vi "calculate_parameters.vi"(10 "Experimental Variables":T2={"Pixel Size before binning (µm)"=14.2, "Imaging Wavelength (m)"=4.61e-07, "Isotope"=84, "1P1 Linewidth (MHz)"=32.0, "Imaging Detuning (MHz)"=0.0, "Software Bin Size"=1, "Exp. Trigger ON time (ms)"=0.0, "Path to spinapi.dll"=path "C:/SpinCore/SpinAPI/lib32/spinapi.dll", "PB clock_freq (MHz)"=100.0} {"Software Bin Size" items=["1"=1, "2"=2, "3"=3, "4"=4, "5"=5, "6"=6, "7"=7, "8"=8]; "Isotope" min=84 max=88; "Imaging Wavelength (m)" format="%#_6p"}) -> (1 "Effective Pixel Size (µm)":dbl, 2 "Cross Section (m^2)":dbl, 3 "Calculated Experimental Values":T1 {"Effective Pixel Size (µm)" format="%#_6p"; "Effective Pixel Area (µm^2)" format="%#_6p"; "Absorption Cross Section (µm)" format="%#_6p"})   [LabVIEW 2016]
uses:
  Controls/ExperimentParameters/experimentalvariables.ctl
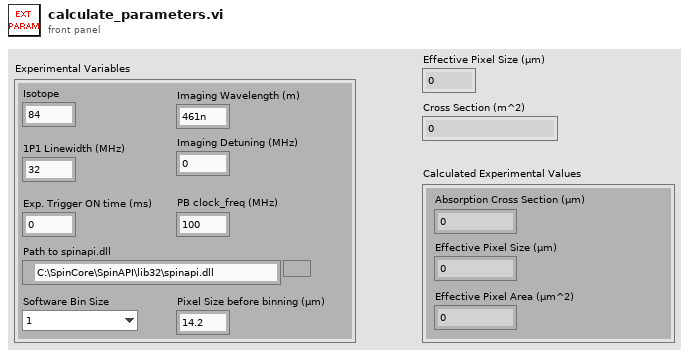
[diagram p1: front panel]
types:
  T1 = cluster{"Absorption Cross Section (µm)":dbl, "Effective Pixel Area (µm^2)":dbl, "Effective Pixel Size (µm)":dbl}
  T2 = typedef "experimentalvariables.ctl" = cluster{"Pixel Size before binning (µm)":dbl, "Imaging Wavelength (m)":dbl, "Isotope":i32, "1P1 Linewidth (MHz)":dbl, "Imaging Detuning (MHz)":dbl, "Software Bin Size":u16, "Exp. Trigger ON time (ms)":dbl, "Path to spinapi.dll":path, "PB clock_freq (MHz)":dbl}
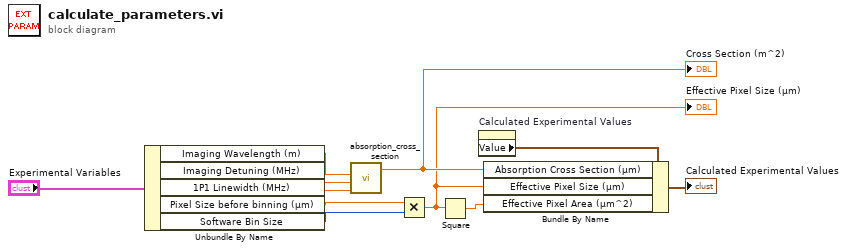
[diagram p0: block diagram]
diagram:
  n1 = Unbundle By Name("Experimental Variables") -> ("Imaging Wavelength (m)"=w10:dbl, "Imaging Detuning (MHz)"=w9:dbl, "1P1 Linewidth (MHz)"=w8:dbl, "Pixel Size before binning (µm)"=w7:dbl, "Software Bin Size"=w2:u16)
  n2 = call "absorption_cross_section.vi"("Linewidth (MHz)"=w8, "Detuning (MHz)"=w9, "Wavelength (m)"=w10) -> ("Cross Section (um^2)"=w4:dbl)  [unwired: 8 in]
  "Cross Section (m^2)" <- w4
  n3 = Multiply(x=w7, y=w2) -> (x*y=w1:dbl)
  "Effective Pixel Size (µm)" <- w1
  n4 = Square(x=w1) -> (x^2=w3:dbl)
  n5 = property on="Calculated Experimental Values" class="Clust (strict)"() -> ("Value"=w5:T1)  [unwired: 2 in, 2 out]
  n6 = Bundle By Name(cluster=w5, "Absorption Cross Section (µm)"=w4, "Effective Pixel Size (µm)"=w1, "Effective Pixel Area (µm^2)"=w3) -> (→"Calculated Experimental Values":T1)
